vi "Read Response.vi"(8 "error in (no error)":errorcluster, 10 "command":u8, 11 "TroSpec in":refnum<class "PL ISTEQ TroSpec.lvclass">) -> (0 "error out":errorcluster, 2 "response payload":u8[](array[numeric]), 3 "TroSpec out":refnum<class "PL ISTEQ TroSpec.lvclass">)   [LabVIEW 2015, in "PL ISTEQ TroSpec.lvclass"]
doc: "Reads device response."
uses:
  PL ISTEQ TroSpec.lvclass
  PL ISTEQ TroSpec.lvclass/PL ISTEQ TroSpec.ctl
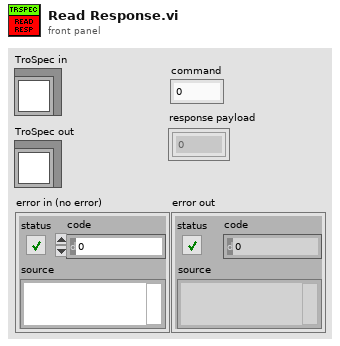
[diagram p1: front panel]
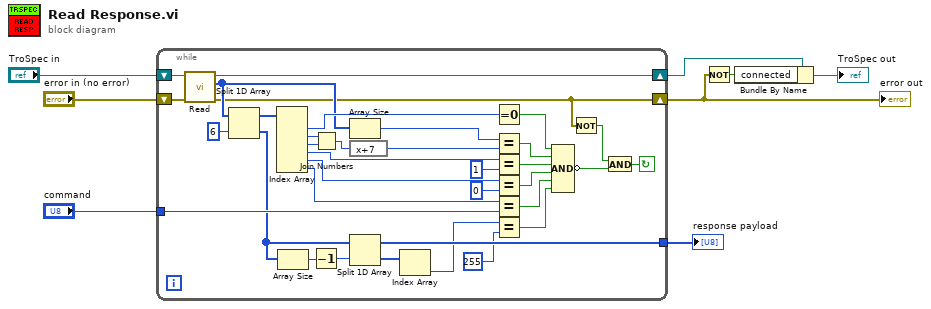
[diagram p0: block diagram]
diagram:
  n1 = while {
    tunnel: [w43] -> w7
    tunnel: "command" -> [w42]
    shift-right: [w28] -> w4
    shift-left: "TroSpec in" -> [w14]
    shift-right: [w11] -> w3
    shift-left: "error in (no error)" -> [w13]
    stop <- w9 continue-if-true
    n2 = call "Read.vi"("error in (no error)"=w13, "TroSpec in"=w14) -> ("error out"=w11:errorcluster, "data"=w21:u8[], "TroSpec out"=w28:refnum<class "PL ISTEQ TroSpec.lvclass">)  [unwired: 7 in]
    n3 = Split 1D Array(array=w21, index=6) -> (first subarray=w27:u8[], second subarray=w26:u8[])
    n4 = Index Array(array=w27) -> (element #1=w39:u8, element #2=w41:u8, element #3=w40:u8, element #4=w25:u8, element #5=w24:u8, element #6=w23:u8)  [unwired: 6 in]
    n5 = Array Size(array=w26) -> (size(s)=w37:i32)
    n6 = Decrement(x=w37) -> (x-1=w36:i32)
    n7 = Join Numbers(hi=w41, lo=w40) -> ((hi.lo)=w19:u16)
    n8 = Array Size(array=w21) -> (size(s)=w20:i32)
    n9 = expression code="x+7"(w19) -> (w18:u16)
    n10 = Split 1D Array(array=w26, index=w36) -> (first subarray=w43:u8[], second subarray=w35:u8[])
    n11 = Index Array(array=w35) -> (element=w33:u8)  [unwired: 1 in]
    n12 = Equal To 0?(x=w39) -> (x = 0?=w17:bool)
    n13 = Equal?(x=w20, y=w18) -> (x = y?=w16:bool)
    n14 = Equal?(x=w25, y=u8 1) -> (x = y?=w31:bool)
    n15 = Equal?(x=w24, y=u8 0) -> (x = y?=w32:bool)
    n16 = Equal?(x=w23, y=w42) -> (x = y?=w30:bool)
    n17 = Equal?(x=w33, y=u8 255 ("command")) -> (x = y?=w29:bool)
    n18 = Compound Arithmetic op=AND(w17, w16, w31, w32, w30, w29) -> (invert w12:bool)
    n19 = Not(x=w11) -> (.not. x?=w10:bool)
    n20 = And(x=w10, y=w12) -> (x .and. y?=w9:bool)
  }
  "error out" <- w3
  "response payload" <- w7
  n21 = Not(x=w3) -> (.not. x?=w5:bool)
  n22 = Bundle By Name(cluster=w4, "connected"=w5) -> (→"TroSpec out":refnum<class "PL ISTEQ TroSpec.lvclass">)
